vi "cRIO_v4.vi"() -> ()   [LabVIEW 2015]
uses:
  <vilib>/FPGAPlugInAG/cRIO-9113/niLvFpga_Open_cRIO-9113.vi
  <vilib>/rvi/interface/common/dynamic/niFpgaDynamicAddResources.vi
  <vilib>/Utility/error.llb/Error Cluster From Error Code.vi
  <vilib>/FPGAPlugInAG/Dynamic/niLvFpga_Run_Dynamic.vi
  <vilib>/rvi/interface/common/niFpgaWaitOnOcc.vi
  <vilib>/rvi/errors/niLvFpgaAdjustHostInterfaceError.vi
  <vilib>/FPGAPlugInAG/Dynamic/niLvFpga_Close_Dynamic.vi
  <vilib>/rvi/interface/nirviOpenFPGA/nirviOpenFPGA.xnode
  FPGA Bitfiles/DW40ticks_FPGATarget_Fpgav4_sI8je36Bpvc.lvbitx
  Fpga_v4.vi
  <vilib>/rvi/interface/nirviMethod/nirviMethod.xnode
  <vilib>/rvi/interface/nirviReadWriteControl/nirviReadWriteControl.xnode
  <vilib>/rvi/interface/nirviCloseFPGA/nirviCloseFPGA.xnode
  <vilib>/rvi/errors/niLvFpgaMergeErrorWithErrorCode.vi
  <vilib>/FPGAPlugInAG/Dynamic/niLvFpga_ReadFifo_Dynamic.vi
  <vilib>/rvi/interface/Simulation/niFpgaSimulationCallBeginRW.vi
  NiFpgaLv.dll
  <vilib>/FPGAPlugInAG/Dynamic/niLvFpga_StartFifo_Dynamic.vi
  <vilib>/FPGAPlugInAG/Dynamic/niLvFpga_ConfigureFifo_Dynamic.vi
panel:
  out "Waveform Graph":u32[](graph)
  out "error out":errorcluster
  out "Actual Depth of FIFO":u32
  out "Initial write Elements Remaining":u32
  in  "stop":bool
  out "Timed Out?":bool
  out "Number of times timed out":u8
  out "backlog (Elements remaing on the write)":u32
  in  "Data write ON/OFF":bool
  out "Time(ms) for a loop":u32
  in  "Stop fpga":bool
  out "x-y 3":u32
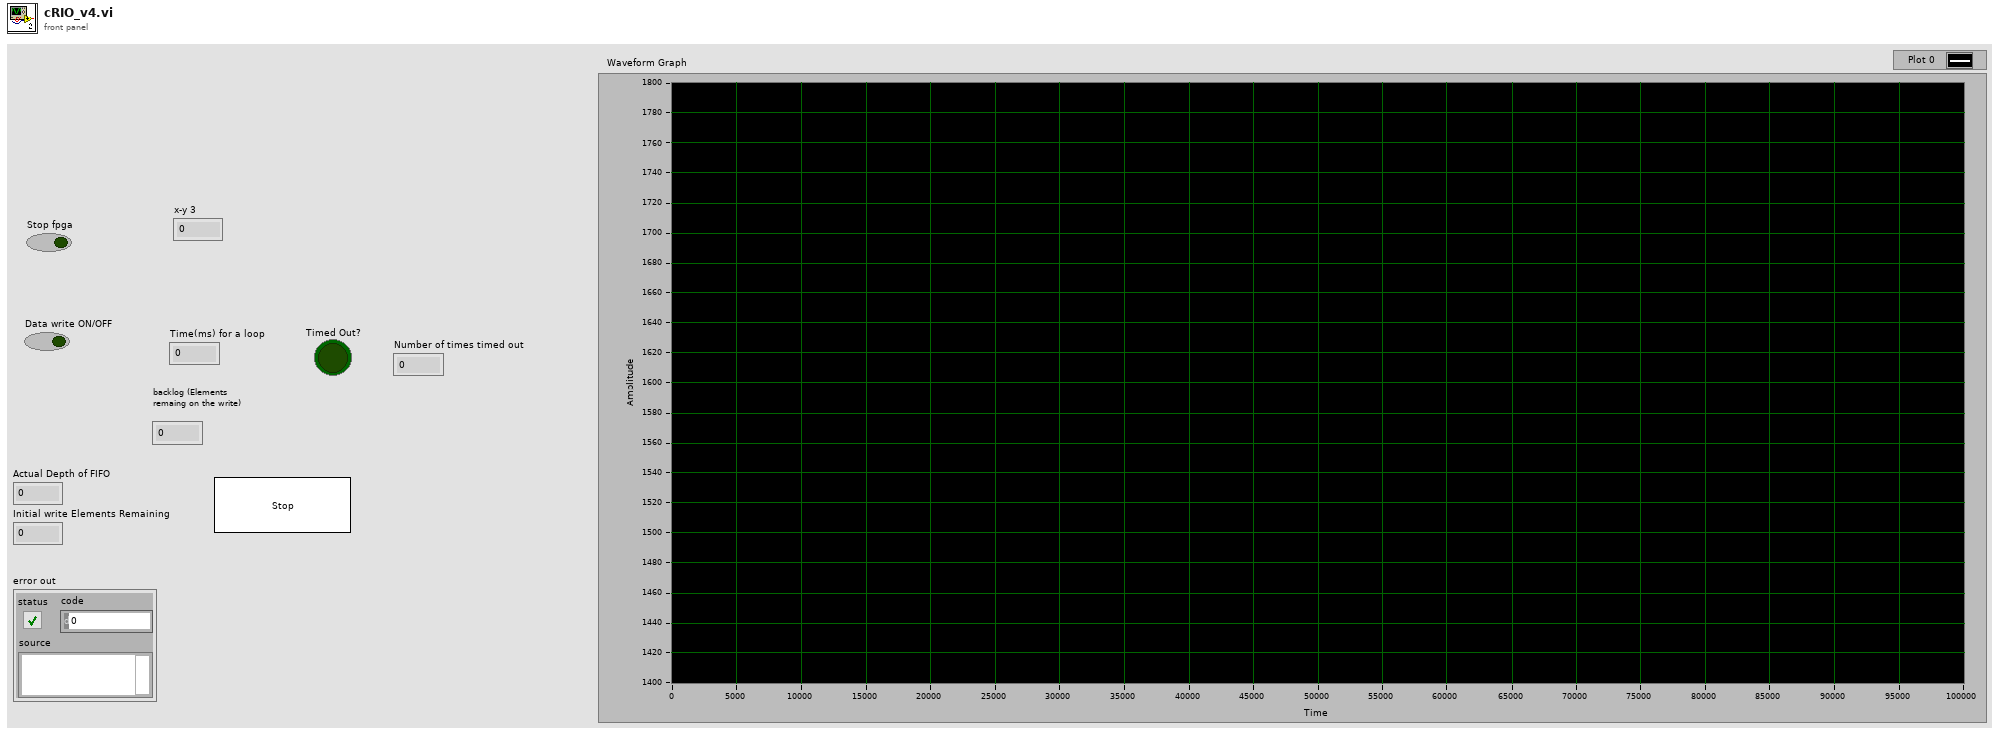
[diagram p1: front panel]
types:
  T1 = enum16{"open", "open or create", "create or replace", "create", "open (read-only)"}
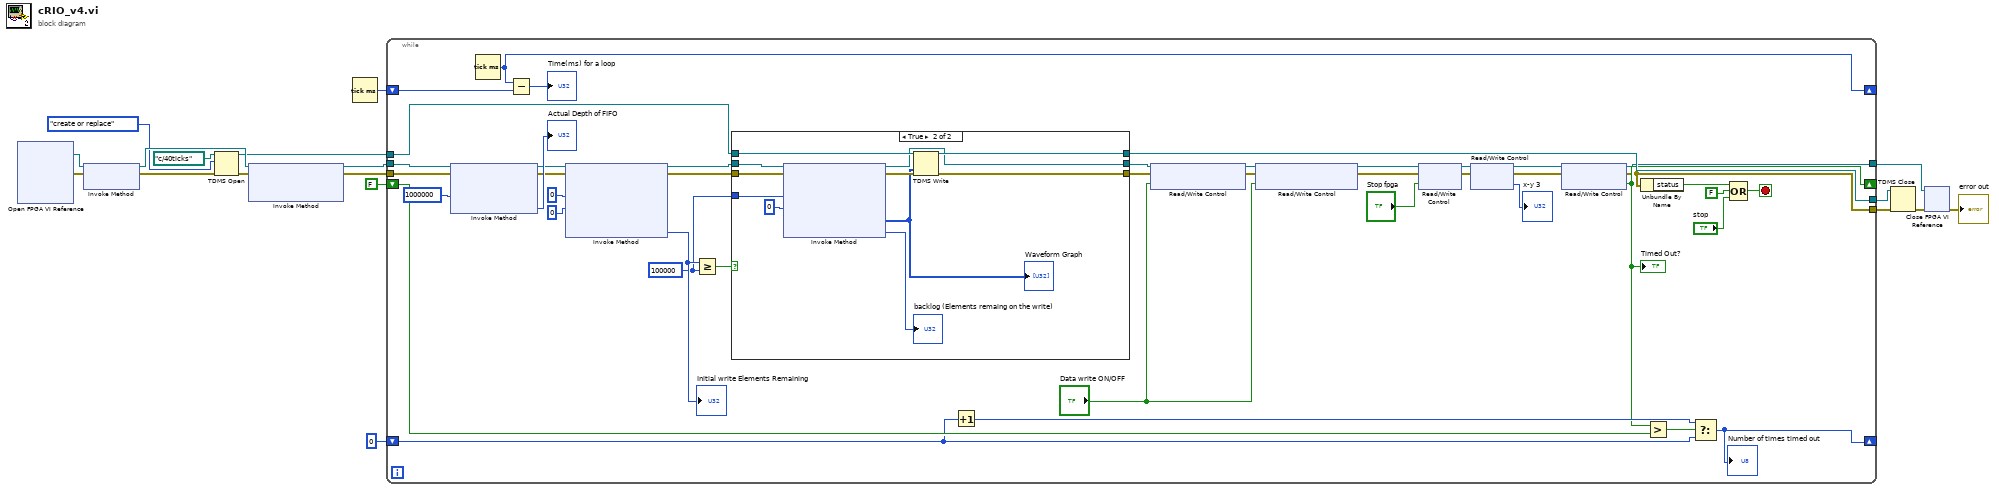
[diagram p0: block diagram]
diagram:
  n1 = xnode "Open FPGA VI Reference"() -> ("FPGA VI Reference Out"=w1:refnum<k20>, "error out"=w2:errorcluster)  [unwired: 2 in]
  n2 = xnode "Invoke Method"("FPGA VI Reference In"=w1, "error in"=w2) -> ("FPGA VI Reference Out"=w17:refnum<k20>, "error out"=w18:errorcluster)
  n3 = TDMS Open(8:w18, 10:T1."create or replace" ("operation (0:open)"), 11:path "c:/40ticks" ("file path")) -> (0:w16:errorcluster, 3:w11:refnum<k34>)  [unwired: 4 in]
  n4 = xnode "Invoke Method"("FPGA VI Reference In"=w17, "error in"=w16) -> ("FPGA VI Reference Out"=w15:refnum<k20>, "error out"=w14:errorcluster)  [unwired: 1 in]
  n5 = Tick Count (ms)() -> (millisecond timer value=w3:u32)
  n6 = while {
    tunnel: w15 -> [w61]
    tunnel: w14 -> [w60]
    tunnel: w11 -> [w52]
    tunnel: [w50] -> w9
    shift-right: [w36] -> _
    shift-left: FALSE ("Timed Out?") -> [w48]
    shift-right: [w44] -> _
    shift-left: u8 0 -> [w46]
    tunnel: [w31] -> w5
    tunnel: [w30] -> w4
    shift-right: [w34] -> _
    shift-left: w3 -> [w35]
    stop <- w49 stop-if-true
    w39 = u32 100000 ("y")
    n7 = xnode "Invoke Method"("FPGA VI Reference In"=w61, "error in"=w60, "Requested Depth"=u32 1000000) -> ("FPGA VI Reference Out"=w57:refnum<k20>, "error out"=w56:errorcluster, "Actual Depth"=→"Actual Depth of FIFO":u32)
    n8 = Tick Count (ms)() -> (millisecond timer value=w34:u32)
    n9 = Subtract(x=w34, y=w35) -> (x-y=→"Time(ms) for a loop":u32)
    n10 = xnode "Invoke Method"("FPGA VI Reference In"=w57, "error in"=w56, "Number of Elements"=u32 0, "Timeout (ms)"=0) -> ("FPGA VI Reference Out"=w40:refnum<k20>, "error out"=w53:errorcluster, "Elements Remaining"=w41:u32)  [unwired: 1 out]
    "Initial write Elements Remaining" <- w41
    n11 = Greater Or Equal?(x=w41, y=w39) -> (x >= y?=w42:bool)
    n12 = case shown="True" w42 {
      tunnel: w53 -> [w62 w71]
      tunnel: w52 -> [w64 w75]
      tunnel: [w62 w74] -> w37
      tunnel: [w64 w73] -> w50
      tunnel: w40 -> [w63 w72]
      tunnel: [w63 w70] -> w38
      tunnel: w39 -> [_ w68]
      frame False {
      }
      frame True {
        n13 = xnode "Invoke Method"("FPGA VI Reference In"=w72, "error in"=w71, "Number of Elements"=w68, "Timeout (ms)"=0) -> ("FPGA VI Reference Out"=w70:refnum<k20>, "error out"=w69:errorcluster, "Data"=w65:u32[], "Elements Remaining"=→"backlog (Elements remaing on the write)":u32)
        "Waveform Graph" <- w65
        n14 = TDMS Write(0:w75, 9:w65, 11:w69) -> (4:w73:refnum<k34>, 15:w74:errorcluster)  [unwired: 3 in, 2 out]
      }
    }
    n15 = Increment(x=w46) -> (x+1=w45:u8)
    n16 = xnode "Read/Write Control"("FPGA VI Reference In"=w38, "error in"=w37, "Data write ON/OFF"="Data write ON/OFF") -> ("FPGA VI Reference Out"=w23:refnum<k20>, "error out"=w22:errorcluster)
    n17 = xnode "Read/Write Control"("FPGA VI Reference In"=w23, "error in"=w22, "Data write ON/OFF 2"="Data write ON/OFF") -> ("FPGA VI Reference Out"=w21:refnum<k20>, "error out"=w20:errorcluster)
    n18 = xnode "Read/Write Control"("FPGA VI Reference In"=w21, "error in"=w20, "stop"="Stop fpga") -> ("FPGA VI Reference Out"=w28:refnum<k20>, "error out"=w27:errorcluster)
    n19 = xnode "Read/Write Control"("FPGA VI Reference In"=w28, "error in"=w27) -> ("FPGA VI Reference Out"=w25:refnum<k20>, "error out"=w26:errorcluster, "x-y 3"=→"x-y 3":u32)
    n20 = xnode "Read/Write Control"("FPGA VI Reference In"=w25, "error in"=w26) -> ("FPGA VI Reference Out"=w31:refnum<k20>, "error out"=w30:errorcluster, "Timed Out?"=w36:bool)
    "Timed Out?" <- w36
    n21 = Unbundle By Name(w30) -> ("status"=w43:bool)
    n22 = Greater?(x=w36, y=w48) -> (0:w47:bool)
    n23 = Select(t=w45, s=w47, f=w46) -> (s? t:f=w44:u8)
    "Number of times timed out" <- w44
    n24 = Compound Arithmetic op=OR(w43, FALSE ("value"), "stop") -> (w49:bool)
  }
  n25 = TDMS Close(8:w4, 11:w9) -> (0:w10:errorcluster)  [unwired: 1 out]
  n26 = xnode "Close FPGA VI Reference"("FPGA VI Reference In"=w5, "error in"=w10) -> ("error out"=→"error out":errorcluster)
